vi "List_files_in_order_of_age.vi"(6 "Files to Hide":string[](array[string]), 7 "wildcardPattern":string, 11 "Folder":path) -> (1 "file names":string[](array[string]))   [LabVIEW 2021]
uses:
  58ee778a-5d97-f040-badd-2762f77315a6.vi
  <vilib>/Comparison/Less/Less Functor/Less Functor.lvclass
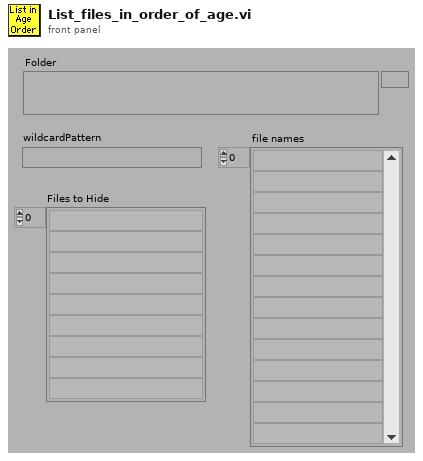
[diagram p1: front panel]
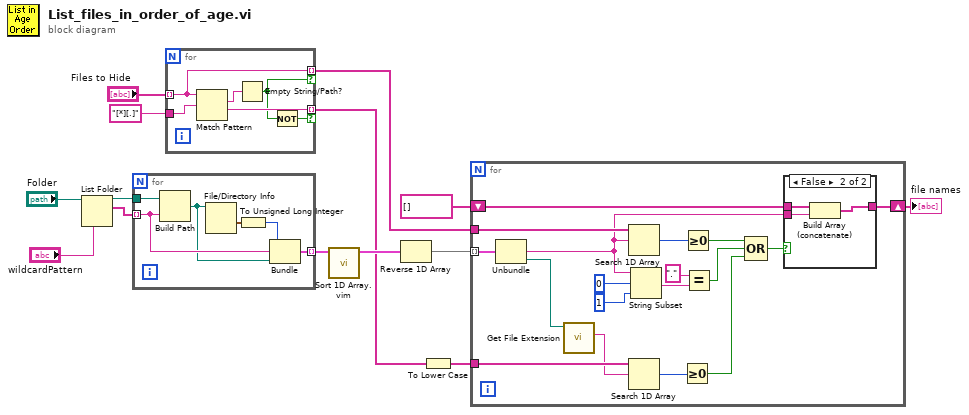
[diagram p0: block diagram]
diagram:
  n1 = List Folder(path="Folder", pattern="wildcardPattern") -> (path out=w14:path, filenames=w13:string[])  [unwired: 1 in, 3 out]
  n2 = for {
    tunnel: w14 -> [w20]
    tunnel: w13 -> [w17] mode=indexing
    tunnel: [w16] -> w9 mode=indexing
    n3 = Build Path(base path=w20, name or relative path=w17) -> (appended path=w15:path)
    n4 = File/Directory Info(path=w15) -> (last mod=w19:timestamp)  [unwired: 1 in, 6 out]
    n5 = To Unsigned Long Integer(number=w19) -> (unsigned 32bit integer=w18:u32)
    n6 = Bundle(w18, w17, "appended path"=w15) -> (w16:cluster{u32, string, "appended path":path})  [unwired: 1 in]
  }
  n7 = for {
    tunnel: "Files to Hide" -> [w26] mode=indexing
    tunnel: [w24] -> w3 mode=indexing if=w21
    tunnel: [w26] -> w5 mode=indexing if=w22
    tunnel: "[*][.]" ("regular expression") -> [w25]
    n8 = Match Pattern(string=w26, regular expression=w25) -> (match substring=w23:string, after substring=w24:string)  [unwired: 1 in, 2 out]
    n9 = Empty String/Path?(string/path=w23) -> (empty?=w22:bool)
    n10 = Not(x=w22) -> (.not. x?=w21:bool)
  }
  n11 = call "Sort 1D Array.vim"("unsorted array"=w9) -> ("sorted array"=w8:cluster{u32, string, "appended path":path}[])  [unwired: 10 in]
  n12 = Reverse 1D Array(array=w8) -> (reversed array=w2:cluster{u32, string, "appended path":path}[])
  n13 = To Lower Case(string=w3) -> (all lower case string=w7:string[])
  n14 = for {
    shift-right: [w42] -> w11
    shift-left: string[] [] -> [w44]
    tunnel: w2 -> [w34] mode=indexing
    tunnel: w5 -> [w43]
    tunnel: w7 -> [w30]
    n15 = Unbundle(w34) -> (w32:string, "appended path"=w31:path)  [unwired: 1 out]
    n16 = call <vilib>:"Get File Extension.vi"("file"=w31) -> ("lowercase file extension"=w29:string)  [unwired: 6 in, 4 out]
    n17 = Search 1D Array(1D array=w43, element=w32) -> (index of element=w41:i32)  [unwired: 1 out]
    n18 = Search 1D Array(1D array=w30, element=w29) -> (index of element=w28:i32)  [unwired: 1 out]
    n19 = String Subset(string=w32, offset (0)=0, length (rest)=1 ("length")) -> (substring=w39:string)
    n20 = Greater Or Equal To 0?(x=w28) -> (x >= 0?=w27:bool)
    n21 = Greater Or Equal To 0?(x=w41) -> (x >= 0?=w36:bool)
    n22 = Equal?(x=".", y=w39) -> (x = y?=w33:bool)
    n23 = Compound Arithmetic op=OR(w36, w33, w27) -> (w35:bool)
    n24 = case shown="False" w35 {
      tunnel: w44 -> [w45 w48]
      tunnel: [w45 w47] -> w42
      tunnel: w32 -> [_ w46]
      frame True {
      }
      frame False {
        n25 = Build Array (concatenate)(w48, w46) -> (w47:string[])
      }
    }
  }
  "file names" <- w11
